vi "Register Observer.vi"(8 "error in (no error)":errorcluster, 10 "Actor Framework.lvlib:Message Enqueuer":refnum<class "Message Enqueuer.lvclass">, 11 "Subject in":refnum<class "Subject.lvclass">) -> (0 "error out":errorcluster, 3 "Subject out":refnum<class "Subject.lvclass">)   [LabVIEW 2013, in "Observer Pattern Actor Interface.lvlib" / "Subject.lvclass"]
uses:
  Subject.lvclass
  <vilib>/ActorFramework/Message Enqueuer/Message Enqueuer.lvclass
  Subject.lvclass/Subject.ctl
  Global 2.vi
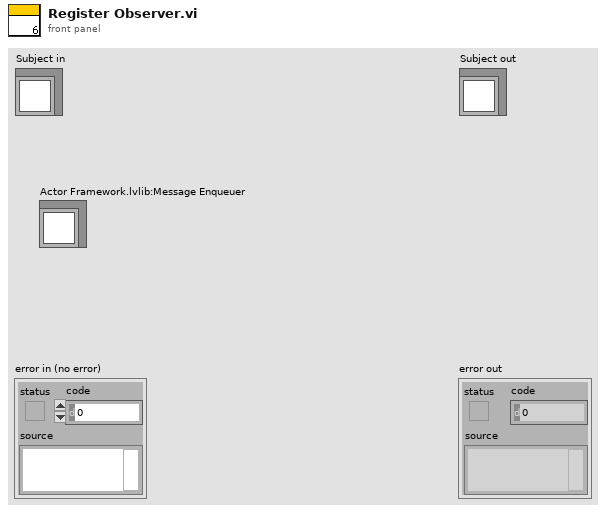
[diagram p1: front panel]
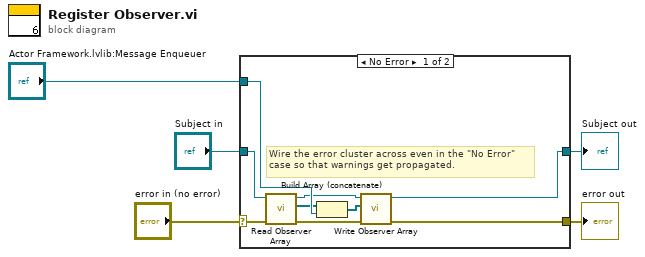
[diagram p0: block diagram]
diagram:
  n1 = case shown="No Error" "error in (no error)" {
    selector: "error in (no error)" -> [w8 w16]
    tunnel: [w7 w16] -> w4
    tunnel: [w10 w15] -> w2
    tunnel: "Subject in" -> [w13 w15]
    tunnel: "Actor Framework.lvlib:Message Enqueuer" -> [w14 _]
    frame No Error {
      # "Wire the error cluster across even in the \"No Error\"\ncase so that warnings get propagated."
      n2 = call "Read Observer Array.vi"("error in (no error)"=w8, "Subject in"=w13) -> ("error out"=w9:errorcluster, "Observer Array"=w12:refnum<class "Message Enqueuer.lvclass">[], "Subject out"=w11:refnum<class "Subject.lvclass">)  [unwired: 7 in]
      n3 = Build Array (concatenate)(w12, w14) -> (w6:refnum<class "Message Enqueuer.lvclass">[])
      n4 = call "Write Observer Array.vi"("error in (no error)"=w9, "Observer Array"=w6, "Subject in"=w11) -> ("error out"=w7:errorcluster, "Subject out"=w10:refnum<class "Subject.lvclass">)  [unwired: 7 in]
    }
    frame Error {
    }
  }
  "error out" <- w4
  "Subject out" <- w2
